vi "Hangup Main.vi"() -> ()   [LabVIEW 2020, in "Hangup Check.lvlib"]
uses:
  Hangup Check.lvlib
  HangupSettings.ctl
  Visualisierungs Elemente/Auswahlfeld.ctl
  AktionFGV Hangup.ctl
  Seiten/FT-IR/FGV FT-IR Gasliste Aktionen.ctl
  Seiten/CalGas Aufschaltung/FGV CalGas Aktionen.ctl
  Sprachverwaltung/FGV Aktion Tabelle zerlegen.ctl
  Messdaten/Aktionen FGV Messdaten.ctl
  Aktion Hangup Test.ctl
  O2 Dichtheitstest/Aktion FGV O2 Leak.ctl
  Funktionstasten/Funktionstasten-Aktion.ctl
  Funktionstasten/Zustaende.ctl
  Seiten/FT-IR/FGV FT-IR Parameter.vi
  Allgemein/allgemeine Sub-VIs.lvlib
  Seiten/FT-IR/FT-IR.lvlib
  Seiten/Grafik/Grafik.lvlib
  Messdaten/Messdaten.lvlib
  Funktionstasten/Funktionstasten.lvlib
  Seiten/CalGas Aufschaltung/CalGas Aufschaltung.lvlib
  O2 Dichtheitstest/O2 Dichtheitstest.lvlib
  Linearisierung V2/Protokoll/Protokoll.lvlib
  Sprachverwaltung/Sprachverwaltung.lvlib
panel:
  out "ppmC1":sgl caption="Ergebnis:" format="%#.1f"
  out "Index":i32
  out "FID":sgl caption="ppmC3" format="%.1f"
  out "Graph CH4":waveform(dbl)(graph)
  out "Bestanden":bool caption="Boolesch"
  out "Zeit":sgl caption="s"
  in  "Textname:":string
  in  "Pfad:":path=path "D:/IAG_Data/Log"
  in  "Speichern":bool
  out "ppmC3":sgl caption="Ergebnis:" format="%#.1f"
  in  "Hangup Settings":T1 {"Grenzwert: C1" format="%#.1f"; "Spankonzentration [ppm]" format="%#.1f"; "Messbereich" items=["---", "0-500", "0-5000", "0-10000"]; "Grenze" items=["Manuell", "Auto"]; "Grenzwert:" format="%#.1f"; "Grenzwert manuell:" format="%#.1f"; "Datenerfassungszeit:" format="%#.1f"; "Nullgas Aufschaltzeit:" format="%#.1f"; "Spangas Aufschaltzeit:" format="%#.1f"; "Aufschaltpunkt" items=["Filterblock", "Analyzer directly", "PNS", "Samplepoint"]; "Kalibriergas" items=["Nitrogen", "Span 1", "Span 2", "Span 3"]}
  in  "Abbrechen":bool
  in  "Test Start":bool
  out "Status":string
  # "Protokoll"
  # "Ergebnis"
  # "Test - Sequenz"
  # "Einstellungen"
  # "Hang-Up-Check"
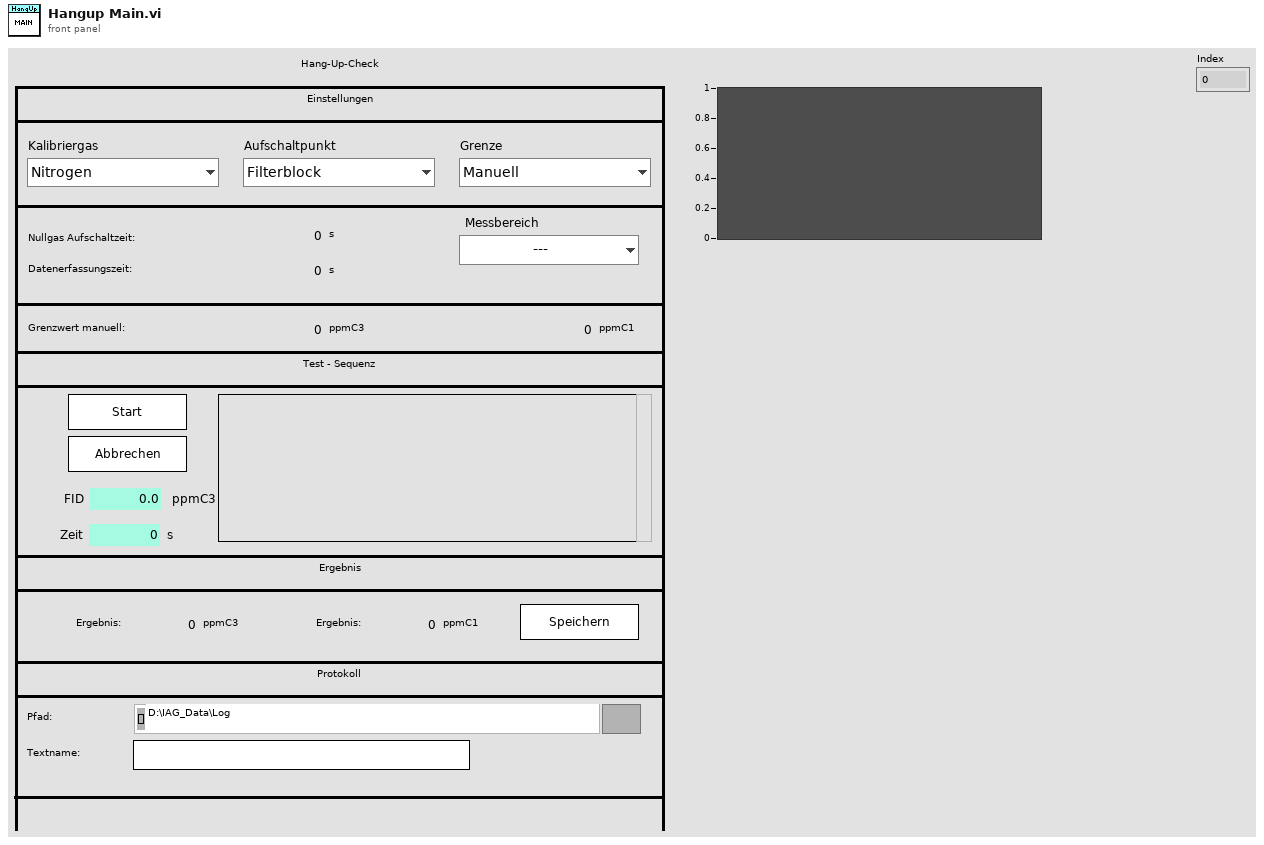
[diagram p1: front panel]
types:
  T1 = typedef "Hangup Check.lvlib/HangupSettings.ctl" = cluster{"Kalibriergas":T2, "Aufschaltpunkt":T2, "Spangas Aufschaltzeit:":sgl, "Nullgas Aufschaltzeit:":sgl, "Datenerfassungszeit:":sgl, "Grenzwert manuell:":sgl, "Grenzwert:":sgl, "Grenze":T2, "Messbereich":T2, "Spankonzentration [ppm]":sgl, "Grenzwert: C1":sgl}
  T2 = typedef "Auswahlfeld.ctl" = u16
  T3 = typedef "Sprachverwaltung.lvlib/FGV Aktion Tabelle zerlegen.ctl" = enum16{"laden", "vereinzeln", "speichern"}
  T4 = typedef "CalGas Aufschaltung.lvlib/FGV CalGas Aktionen.ctl" = enum16{"lesen", "Analysator Auswahl", "Def.CalGas", "Aufschaltung CalGas", "laden", "speichern", "KAL extrahieren"}
  T5 = typedef "FT-IR.lvlib/FGV FT-IR Gasliste Aktionen.ctl" = enum16{"lesen", "Gasliste FT-IR", "Gasliste ausgelesen", "laden", "speichern", "löschen"}
  T6 = enum8{"Enabled", "Disabled", "Disabled and Grayed Out"}
  T7 = typedef "Hangup Check.lvlib/AktionFGV Hangup.ctl" = enum16{"lesen", "Hangup Settings", "Protokoll", "Pfad", "laden", "speichern"}
  T8 = typedef "String - Ausgabefeld.ctl" = string
  T9 = typedef "CalGas Aufschaltung.lvlib/Definition CalGas Anzeige.ctl" = cluster{"Namen":T10, "Werte":T12, "Werte 2":T12, "Einheit":T14, "Messbereiche":T15}
  T10 = typedef "CalGas Aufschaltung.lvlib/CalGas-Namen.ctl" = cluster{"Name":T11, "Name 2":T11, "Name 3":T11, "Name 4":T11, "Name 5":T11, "Name 6":T11, "Name 7":T11, "Name 8":T11, "Name 9":T11, "Name 10":T11, "Name 11":T11, "Name 12":T11}
  T11 = typedef "String - Eingabefeld.ctl" = string
  T12 = typedef "CalGas Aufschaltung.lvlib/CalGas-Werte.ctl" = cluster{"Konzentration 1":T13, "Konzentration 2":T13, "Konzentration 3":T13, "Konzentration 4":T13, "Konzentration 5":T13, "Konzentration 6":T13, "Konzentration 7":T13, "Konzentration 8":T13, "Konzentration 9":T13, "Konzentration 10":T13, "Konzentration 11":T13, "Konzentration 12":T13}
  T13 = typedef "Zahlen-Eingabefeld.ctl" = sgl
  T14 = typedef "CalGas Aufschaltung.lvlib/CalGas-Einheit.ctl" = cluster{"Einheit 1":T2, "Einheit 2":T2, "Einheit 3":T2, "Einheit 4":T2, "Einheit 5":T2, "Einheit 6":T2, "Einheit 7":T2, "Einheit 8":T2, "Einheit 9":T2, "Einheit 10":T2, "Einheit 11":T2, "Einheit 12":T2}
  T15 = typedef "CalGas Aufschaltung.lvlib/CalGas-Messbereiche.ctl" = cluster{"Messbereich 1":T2, "Messbereich 2":T2, "Messbereich 3":T2, "Messbereich 4":T2, "Messbereich 5":T2, "Messbereich 6":T2, "Messbereich 7":T2, "Messbereich 8":T2, "Messbereich 9":T2, "Messbereich 10":T2, "Messbereich 11":T2, "Messbereich 12":T2}
  T16 = typedef "Messdaten.lvlib/Aktionen FGV Messdaten.ctl" = enum16{"lesen", "schreiben", "löschen", "Mittelwerte", "Komponente"}
  T17 = typedef "Hangup Check.lvlib/Aktion Hangup Test.ctl" = enum16{"ini", "0-Gas aufschalten", "warten", "E-Gas aufschalten", "auswerten", "Fertig"}
  T18 = typedef "O2 Dichtheitstest.lvlib/Aktion FGV O2 Leak.ctl" = enum16{"lesen", "O2 settings", "Pfad", "Protokoll", "laden", "speichern"}
  T19 = typedef "Funktionstasten.lvlib/Zustaende.ctl" = enum16{"Standby", "Pause", "Eco", "Messen", "Kalibrieren", "Spülen Filter", "Spülen Leitung", "Umgebungsluft", "0-Gas", "Cal-Gas", "CG zu PNS", "-------------", "Init 1", "Init 2", "Init 3", "Init 4", "Messen vorbereiten", "Messen durchführen", "Exit"}
  T20 = typedef "Funktionstasten.lvlib/Funktionstasten-Aktion.ctl" = enum16{"Initialisieren", "Zustand setzen", "Taste gedrückt", "Fehler speichern", "Lesen", "Manuell", "Remote", "Bitparallel", "Samplepoint", "Zeit Prüfen", "reset Umschalten"}
  T21 = typedef "Hangup Check.lvlib/Protokoll.ctl" = cluster{"FID Mittelwert 0":sgl, "FID Mittelwert E":sgl, "Messgasdruck Amium":sgl, "Startzeit":timestamp, "Endzeit":timestamp, "Bestanden?":bool}
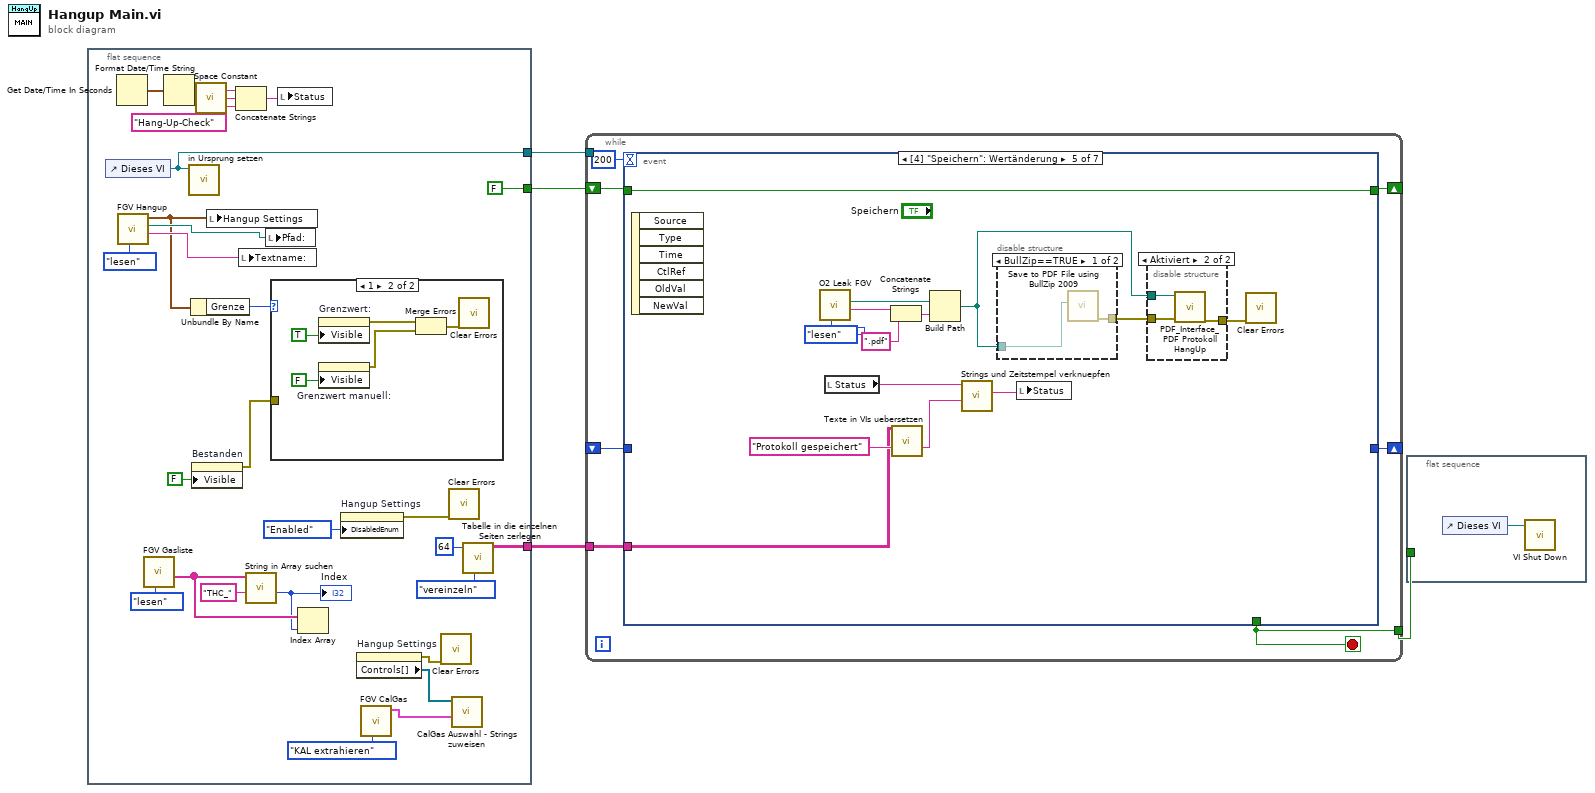
[diagram p0: block diagram]
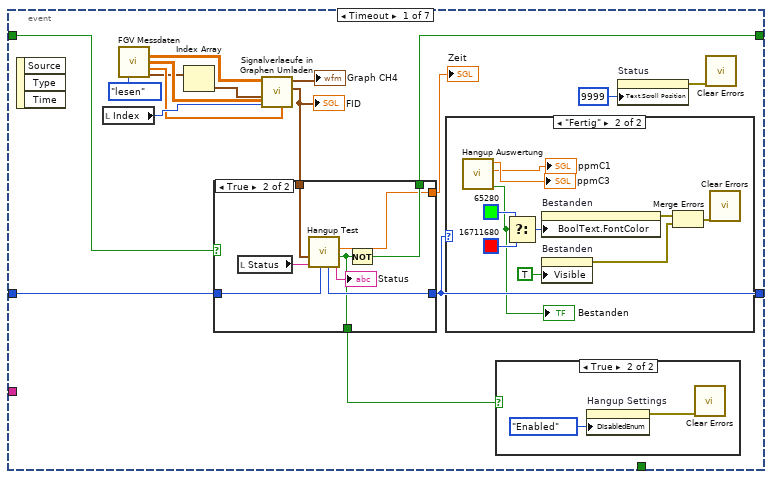
[diagram p2: hidden frame]
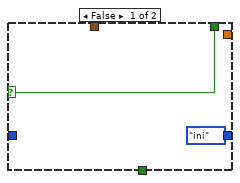
[diagram p5: hidden frame]
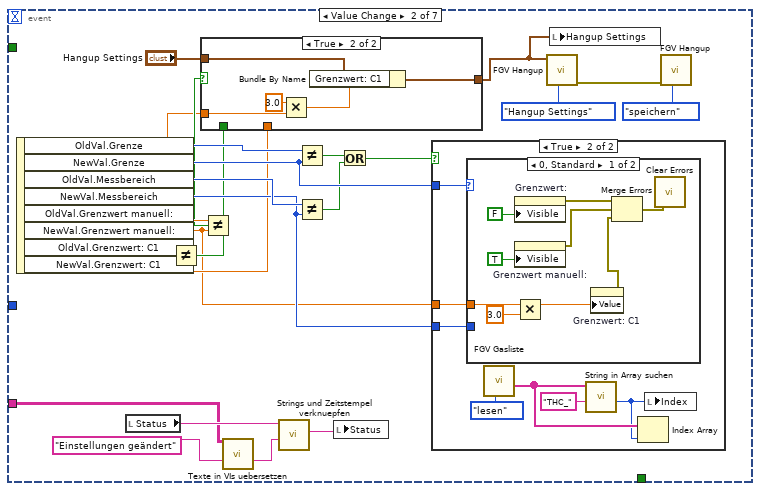
[diagram p6: hidden frame]
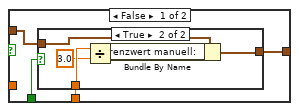
[diagram p7: hidden frame]
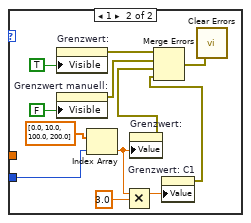
[diagram p10: hidden frame]
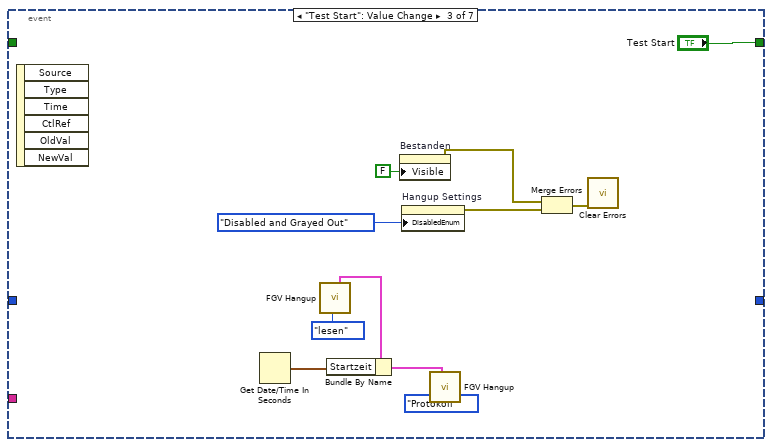
[diagram p11: hidden frame]
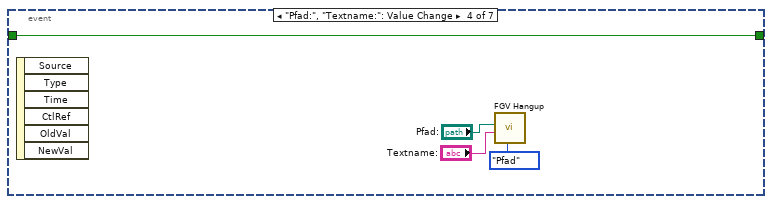
[diagram p12: hidden frame]
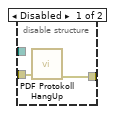
[diagram p13: hidden frame]
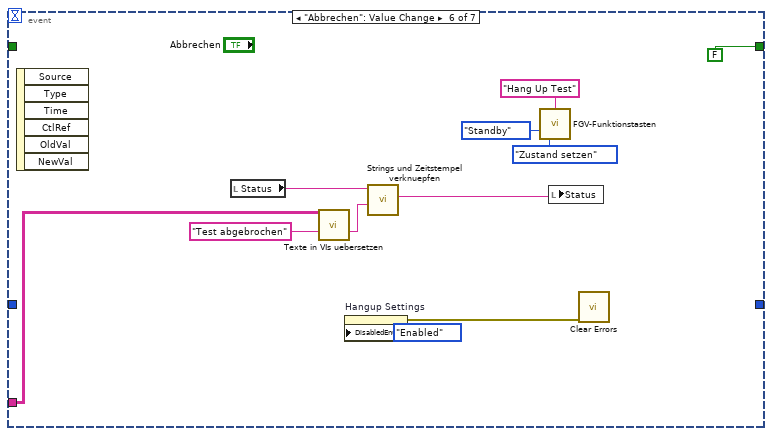
[diagram p15: hidden frame]
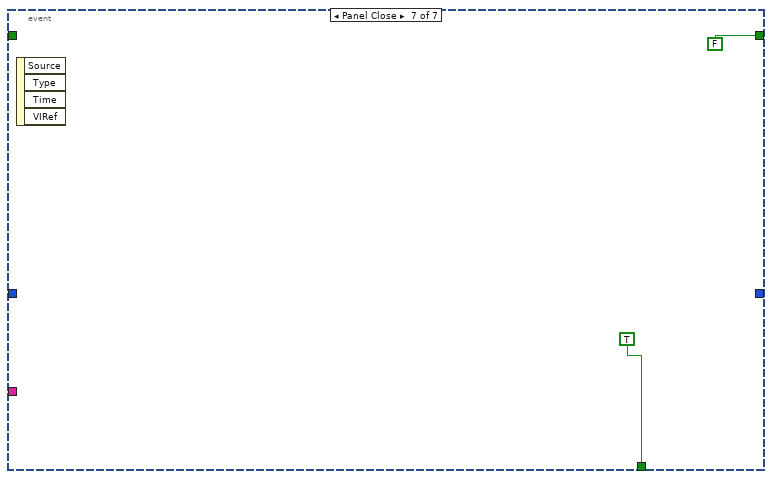
[diagram p16: hidden frame]
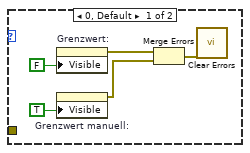
[diagram p17: hidden frame]
diagram:
  n1 = flat-sequence {
    tunnel: [w26] -> w4
    tunnel: [FALSE] -> w2
    tunnel: [w5] -> w1
    frame #0 {
      n2 = control-ref of="Dieses VI"() -> (w26:refnum<vi>)
      n3 = Get Date/Time In Seconds() -> (seconds since 1Jan1904=w22:timestamp)
      n4 = call "FGV Hangup.vi"("Aktion"=AktionFGV_Hangup."lesen") -> ("Textname:"=w29:string, "Pfad:"=w30:path, "Hangup Settings"=w28:T1)  [unwired: 6 in, 2 out]
      n5 = call "FGV Gasliste.vi"("Aktionen"=FGV_FT-IR_Gasliste_Aktionen."lesen") -> ("Aktuelle Gasliste gesamt"=w17:T8[])  [unwired: 8 in, 2 out]
      n6 = Format Date/Time String(seconds (now)=w22) -> (date/time string=w23:string)  [unwired: 2 in]
      n7 = call "in Ursprung setzen.vi"("VI Referenz"=w26) -> ()  [unwired: 10 in, 1 out]
      n8 = Unbundle By Name(w28) -> ("Grenze"=w27:T2)
      n9 = property on="Bestanden" class="Bool. (strikt)"("Visible"=FALSE ("Sichtbar")) -> (error out=w12:errorcluster)  [unwired: 2 in, 1 out]
      n10 = call <vilib>:"Space Constant.vi"() -> ("String"=w24:string)
      n11 = local write "Hangup Settings"(w28) -> ()
      n12 = Concatenate Strings(w23, w24, "Hang-Up-Check" ("String")) -> (w21:string)
      n13 = local write "Textname:"(w29) -> ()
      n14 = call "String in Array suchen.vi"("Nach String/Zeichen suchen (-)"="THC_", "String-Array"=w17) -> ("Index"=w14:i32)  [unwired: 7 in, 2 out]
      "Index" <- w14
      n15 = local write "Pfad:"(w30) -> ()
      n16 = case shown="1" w27 {
        tunnel: w12 -> [_ _]
        frame 0, Default {
          n17 = property on="Grenzwert:" class="DigWert (strikt)"("Visible"=FALSE) -> (error out=w33:errorcluster)  [unwired: 2 in, 1 out]
          n18 = property on="Grenzwert manuell:" class="DigWert (strikt)"("Visible"=TRUE) -> (error out=w32:errorcluster)  [unwired: 2 in, 1 out]
          n19 = Merge Errors(w33, w32) -> (w34:errorcluster)
          n20 = call <vilib>:"Clear Errors.vi"("error in (no error)"=w34) -> ()  [unwired: 5 in, 2 out]
        }
        frame 1 {
          n21 = property on="Grenzwert:" class="DigWert (strikt)"("Visible"=TRUE) -> (error out=w38:errorcluster)  [unwired: 2 in, 1 out]
          n22 = property on="Grenzwert manuell:" class="DigWert (strikt)"("Visible"=FALSE) -> (error out=w37:errorcluster)  [unwired: 2 in, 1 out]
          n23 = Merge Errors(w38, w37) -> (w39:errorcluster)
          n24 = call <vilib>:"Clear Errors.vi"("error in (no error)"=w39) -> ()  [unwired: 5 in, 2 out]
        }
      }
      n25 = local write "Status"(w21) -> ()
      n26 = Index Array(array=w17, index=w14) -> ()  [unwired: 1 out]
      n27 = property on="Hangup Settings" class="Cluster (strikt)"("DisabledEnum"=T6."Enabled" ("Deaktiviert")) -> (error out=w19:errorcluster)  [unwired: 2 in, 1 out]
      n28 = property on="Hangup Settings" class="Cluster (strikt)"() -> (error out=w8:errorcluster, "Controls[]"=w11:refnum<vi>[])  [unwired: 2 in, 1 out]
      n29 = call "FGV CalGas.vi"("Aktionen"=FGV_CalGas_Aktionen."KAL extrahieren") -> ("Def.CalGas"=w10:T9)  [unwired: 6 in, 4 out]
      n30 = call <vilib>:"Clear Errors.vi"("error in (no error)"=w8) -> ()  [unwired: 5 in, 2 out]
      n31 = call <vilib>:"Clear Errors.vi"("error in (no error)"=w19) -> ()  [unwired: 5 in, 2 out]
      n32 = call "CalGas Auswahl - Strings zuweisen.vi"("Def.CalGas"=w10, "Aufschaltung CalGas"=w11) -> ()  [unwired: 9 in, 1 out]
      n33 = call "Tabelle in die einzelnen Seiten zerlegen.vi"("Aktion"=FGV_Aktion_Tabelle_zerlegen."vereinzeln", "Index (Seite)"=64) -> ("Sprachliste"=w5:string[][])  [unwired: 7 in, 2 out]
    }
  }
  n34 = while {
    tunnel: w4 -> [_]
    tunnel: [w48] -> w3
    shift-right: [w47] -> _
    shift-left: w2 -> [w46]
    shift-right: [w44] -> _
    shift-left: _ -> [w43]
    tunnel: w1 -> [w42]
    stop <- w48 stop-if-true
    n35 = event shown="[4] \"Speichern\": Wertänderung" {
      selector: _ -> [_ _ _ _ _ _ _]
      dyn-events: _ -> [_ _ _ _ _ _ _]
      timeout: 200 -> [_ _ _ _ _ _ _]
      tunnel: [_ _ _ _ _ _ TRUE] -> w48
      tunnel: [w61 _ "Test Start" w165 w180 FALSE ("Test Start") FALSE ("Test Start")] -> w47
      tunnel: w46 -> [w63 _ _ w165 w180 _ _]
      tunnel: [w58 _ _ _ _ _ _] -> w44
      tunnel: w43 -> [w62 _ _ _ _ _ _]
      tunnel: w42 -> [_ w88 _ _ w175 w190 _]
      event Timeout {
        n36 = event-data() -> ()  [unwired: 1 in, 3 out]
        n37 = local read "Index"() -> (w57:i32)
        n38 = call "FGV Messdaten.vi"("Aktionen"=Aktionen_FGV_Messdaten."lesen") -> ("Messdaten"=w53:sgl[][], "Mittelwertdaten"=w55:sgl[][], "Deviation"=w56:sgl[], "Zeitstempeln"=w51:timestamp[])  [unwired: 6 in, 5 out]
        n39 = Index Array(array=w51) -> (element=w54:timestamp)  [unwired: 1 in]
        n40 = call "Signalverlaeufe in Graphen Umladen.vi"("Deviation"=w56, "Mittelwertdaten"=w55, "Gas-Auswahl"=w57, "t0"=w54, "Werte"=w53) -> ("Mittelwert"=w49:waveform(dbl), "Waveform"=→"Graph CH4":waveform(dbl))  [unwired: 2 in, 3 out]
        "FID" <- w49
        n41 = case shown="True" w63 {
          selector: w63 -> [w78 _]
          tunnel: [Aktion_Hangup_Test."ini" ("Aktion Hangup Test 2") w87] -> w58
          tunnel: w62 -> [_ w86]
          tunnel: [w78 w85] -> w61
          tunnel: [_ w82] -> w60
          tunnel: [_ w81] -> w59
          tunnel: w49 -> [_ w80]
          frame False {
          }
          frame True {
            n42 = local read "Status"() -> (w83:string)
            n43 = call "Hangup Test.vi"("Aktion Hangup Test"=w86, "Status"=w83, "FID"=w80) -> ("Status"=→"Status":string, "Test beendet?"=w82:bool, "countdonw"=w81:dbl, "Aktion Hangup Test 2"=w87:T17)  [unwired: 5 in]
            n44 = Not(x=w82) -> (.not. x?=w85:bool)
          }
        }
        "Zeit" <- w59
        n45 = case shown="\"Fertig\"" w58 {
          frame "ini", Default {
          }
          frame "Fertig" {
            n46 = call "Hangup Auswertung.vi"() -> ("Bestanden"=w67:bool, "Ergebnis ppmC1 2"=→"ppmC1":sgl, "Ergebnis ppmC3"=→"ppmC3":sgl)  [unwired: 9 in]
            "Bestanden" <- w67
            n47 = Select(t=u32 65280, s=w67, f=u32 16711680) -> (s? t:f=w73:u32)
            n48 = property on="Bestanden" class="Bool. (strikt)"("BoolText.FontColor"=w73) -> (error out=w70:errorcluster)  [unwired: 2 in, 1 out]
            n49 = property on="Bestanden" class="Bool. (strikt)"("Visible"=TRUE ("Sichtbar")) -> (error out=w71:errorcluster)  [unwired: 2 in, 1 out]
            n50 = Merge Errors(w70, w71) -> (w69:errorcluster)
            n51 = call <vilib>:"Clear Errors.vi"("error in (no error)"=w69) -> ()  [unwired: 5 in, 2 out]
          }
        }
        n52 = case shown="True" w60 {
          frame False {
          }
          frame True {
            n53 = property on="Hangup Settings" class="Cluster (strikt)"("DisabledEnum"=T6."Enabled" ("Deaktiviert")) -> (error out=w76:errorcluster)  [unwired: 2 in, 1 out]
            n54 = call <vilib>:"Clear Errors.vi"("error in (no error)"=w76) -> ()  [unwired: 5 in, 2 out]
          }
        }
        n55 = property on="Status" class="Str"("Text.Scroll Position"=u32 9999 ("Text.Anzeigeposition")) -> (error out=w64:errorcluster)  [unwired: 2 in, 1 out]
        n56 = call <vilib>:"Clear Errors.vi"("error in (no error)"=w64) -> ()  [unwired: 5 in, 2 out]
      }
      event Value Change {
        n57 = event-data() -> ("OldVal.Grenze"=w105:T2, "NewVal.Grenze"=w104:T2, "OldVal.Messbereich"=w103:T2, "NewVal.Messbereich"=w99:T2, "OldVal.Grenzwert manuell:"=w98:sgl, "NewVal.Grenzwert manuell:"=w91:sgl, "OldVal.Grenzwert: C1"=w97:sgl, "NewVal.Grenzwert: C1"=w93:sgl)  [unwired: 1 in]
        n58 = local read "Status"() -> (w107:string)
        n59 = Not Equal?(x=w97, y=w93) -> (x != y?=w94:bool)
        n60 = Not Equal?(x=w98, y=w91) -> (x != y?=w95:bool)
        n61 = case shown="True" w95 {
          tunnel: "Hangup Settings" -> [w112 w125]
          tunnel: [w111 w124] -> w92
          tunnel: w91 -> [_ w123]
          tunnel: w94 -> [w114 _]
          tunnel: w93 -> [w113 _]
          frame False {
            n62 = case shown="True" w114 {
              tunnel: w113 -> [_ w120]
              tunnel: w112 -> [w115 w117]
              tunnel: [w115 w116] -> w111
              frame False {
              }
              frame True {
                n63 = Divide(x=w120, y=sgl 3.0) -> (x/y=w118:sgl)
                n64 = Bundle By Name(cluster=w117, "Grenzwert manuell:"=w118) -> (w116:T1)
              }
            }
          }
          frame True {
            n65 = Multiply(x=sgl 3.0, y=w123) -> (x*y=w121:sgl)
            n66 = Bundle By Name(cluster=w125, "Grenzwert: C1"=w121) -> (w124:T1)
          }
        }
        n67 = call "Texte in VIs uebersetzen.vi"("Sprachliste"=w88, "String zum Übersetzen"="Einstellungen geändert" ("String 1 hinzufügen")) -> ("String zum Übersetzen"=w89:string)  [unwired: 9 in, 4 out]
        n68 = call "Strings und Zeitstempel verknuepfen.vi"("String 1 hinzufügen"=w89, "Eingagns String"=w107) -> ("Verknüpfter String"=w106:string)  [unwired: 9 in]
        n69 = Not Equal?(x=w105, y=w104) -> (x != y?=w102:bool)
        n70 = Not Equal?(x=w103, y=w99) -> (x != y?=w101:bool)
        n71 = local write "Status"(w106) -> ()
        n72 = Or(x=w102, y=w101) -> (x .or. y?=w100:bool)
        n73 = case shown="True" w100 {
          tunnel: w104 -> [_ w132]
          tunnel: w99 -> [_ w127]
          tunnel: w91 -> [_ w126]
          frame False {
          }
          frame True {
            n74 = case shown="0, Standard" w132 {
              tunnel: w127 -> [_ w146]
              tunnel: w126 -> [w135 _]
              frame 0, Default {
                n75 = property on="Grenzwert:" class="DigWert (strikt)"("Visible"=FALSE) -> (error out=w138:errorcluster)  [unwired: 2 in, 1 out]
                n76 = property on="Grenzwert manuell:" class="DigWert (strikt)"("Visible"=TRUE) -> (error out=w137:errorcluster)  [unwired: 2 in, 1 out]
                n77 = Multiply(x=w135, y=sgl 3.0) -> (x*y=w134:sgl)
                n78 = property on="Grenzwert: C1" class="DigWert (strikt)"("Value"=w134) -> (error out=w136:errorcluster)  [unwired: 2 in, 1 out]
                n79 = Merge Errors(w138, w137, w136) -> (w139:errorcluster)
                n80 = call <vilib>:"Clear Errors.vi"("error in (no error)"=w139) -> ()  [unwired: 5 in, 2 out]
              }
              frame 1 {
                n81 = property on="Grenzwert:" class="DigWert (strikt)"("Visible"=TRUE) -> (error out=w150:errorcluster)  [unwired: 2 in, 1 out]
                n82 = property on="Grenzwert manuell:" class="DigWert (strikt)"("Visible"=FALSE) -> (error out=w149:errorcluster)  [unwired: 2 in, 1 out]
                n83 = Index Array(array=sgl[] [0.0, 10.0, 100.0, 200.0] ("Wert"), index=w146) -> (element=w145:sgl)
                n84 = Multiply(x=w145, y=sgl 3.0) -> (x*y=w144:sgl)
                n85 = property on="Grenzwert:" class="DigWert (strikt)"("Value"=w145) -> (error out=w148:errorcluster)  [unwired: 2 in, 1 out]
                n86 = property on="Grenzwert: C1" class="DigWert (strikt)"("Value"=w144) -> (error out=w142:errorcluster)  [unwired: 2 in, 1 out]
                n87 = Merge Errors(w150, w149, w148, w142) -> (w151:errorcluster)
                n88 = call <vilib>:"Clear Errors.vi"("error in (no error)"=w151) -> ()  [unwired: 5 in, 2 out]
              }
            }
            n89 = call "FGV Gasliste.vi"("Aktionen"=FGV_FT-IR_Gasliste_Aktionen."lesen") -> ("Aktuelle Gasliste gesamt"=w129:T8[])  [unwired: 8 in, 2 out]
            n90 = call "String in Array suchen.vi"("Nach String/Zeichen suchen (-)"="THC_", "String-Array"=w129) -> ("Index"=w128:i32)  [unwired: 7 in, 2 out]
            n91 = Index Array(array=w129, index=w128) -> ()  [unwired: 1 out]
            n92 = local write "Index"(w128) -> ()
          }
        }
        n93 = call "FGV Hangup.vi"("Aktion"=AktionFGV_Hangup."Hangup Settings", "Hangup Settings"=w92) -> ("error out"=w108:errorcluster)  [unwired: 5 in, 4 out]
        n94 = local write "Hangup Settings"(w92) -> ()
        n95 = call "FGV Hangup.vi"("Aktion"=AktionFGV_Hangup."speichern", "error in (no error)"=w108) -> ()  [unwired: 5 in, 5 out]
      }
      event "Test Start": Value Change {
        n96 = event-data() -> ()  [unwired: 1 in, 6 out]
        n97 = Get Date/Time In Seconds() -> (seconds since 1Jan1904=w157:timestamp)
        n98 = call "FGV Hangup.vi"("Aktion"=AktionFGV_Hangup."lesen") -> ("Protokoll"=w159:T21)  [unwired: 6 in, 4 out]
        n99 = Bundle By Name(cluster=w159, "Startzeit"=w157) -> (w161:T21)
        n100 = property on="Bestanden" class="Bool. (strikt)"("Visible"=FALSE ("Sichtbar")) -> (error out=w154:errorcluster)  [unwired: 2 in, 1 out]
        n101 = property on="Hangup Settings" class="Cluster (strikt)"("DisabledEnum"=T6."Disabled and Grayed Out" ("Deaktiviert")) -> (error out=w162:errorcluster)  [unwired: 2 in, 1 out]
        n102 = call "FGV Hangup.vi"("Aktion"=AktionFGV_Hangup."Protokoll", "Protokoll"=w161) -> ()  [unwired: 5 in, 5 out]
        n103 = Merge Errors(w154, w162) -> (w155:errorcluster)
        n104 = call <vilib>:"Clear Errors.vi"("error in (no error)"=w155) -> ()  [unwired: 5 in, 2 out]
      }
      event "Pfad:", "Textname:": Value Change {
        n105 = event-data() -> ()  [unwired: 1 in, 6 out]
        n106 = call "FGV Hangup.vi"("Aktion"=AktionFGV_Hangup."Pfad", "Textname:"="Textname:", "Pfad:"="Pfad:") -> ()  [unwired: 4 in, 5 out]
      }
      event "Speichern": Value Change {
        n107 = event-data() -> ()  [unwired: 1 in, 6 out]
        n108 = call "O2 Leak FGV.vi"("Aktion"=Aktion_FGV_O2_Leak."lesen") -> ("Textname:"=w173:string, "Pfad:"=w174:path)  [unwired: 6 in, 3 out]
        n109 = local read "Status"() -> (w182:string)
        n110 = Concatenate Strings(w173, ".pdf") -> (w172:string)
        n111 = call "Texte in VIs uebersetzen.vi"("Sprachliste"=w175, "String zum Übersetzen"="Protokoll gespeichert" ("String 1 hinzufügen")) -> ("String zum Übersetzen"=w176:string)  [unwired: 9 in, 4 out]
        n112 = Build Path(base path=w174, name or relative path=w172) -> (appended path=w169:path)
        n113 = call "Strings und Zeitstempel verknuepfen.vi"("String 1 hinzufügen"=w176, "Eingagns String"=w182) -> ("Verknüpfter String"=w181:string)  [unwired: 9 in]
        n114 = disable-structure shown="BullZip==TRUE" {
          disable-tunnel: [w189 _] -> w178
          disable-tunnel: w169 -> [w188 _]
          frame condition #0 {
            n115 = call "Save to PDF File using BullZip 2009.vi"("Save PDF File Path"=w188) -> ("error out"=w189:errorcluster)  [unwired: 10 in]
          }
          frame condition #1 (active) {
          }
        }
        n116 = local write "Status"(w181) -> ()
        n117 = disable-structure shown="Aktiviert" {
          disable-tunnel: [w184 w186] -> w179
          disable-tunnel: w178 -> [w183 w187]
          disable-tunnel: w169 -> [_ w185]
          frame Disabled {
            n118 = call "PDF Protokoll HangUp.vi"("error in (no error)"=w183) -> ("error out"=w184:errorcluster)  [unwired: 10 in]
          }
          frame Enabled {
            n119 = call "PDF_Interface_PDF Protokoll HangUp.vi"("error in (no error)"=w187, "Save PDF File Path"=w185) -> ("error out"=w186:errorcluster)  [unwired: 9 in]
          }
        }
        n120 = call <vilib>:"Clear Errors.vi"("error in (no error)"=w179) -> ()  [unwired: 5 in, 2 out]
      }
      event "Abbrechen": Value Change {
        n121 = event-data() -> ()  [unwired: 1 in, 6 out]
        n122 = local read "Status"() -> (w199:string)
        n123 = call "Texte in VIs uebersetzen.vi"("Sprachliste"=w190, "String zum Übersetzen"="Test abgebrochen" ("String 1 hinzufügen")) -> ("String zum Übersetzen"=w191:string)  [unwired: 9 in, 4 out]
        n124 = property on="Hangup Settings" class="Cluster (strikt)"("DisabledEnum"=T6."Enabled" ("Deaktiviert")) -> (error out=w196:errorcluster)  [unwired: 2 in, 1 out]
        n125 = call "Strings und Zeitstempel verknuepfen.vi"("String 1 hinzufügen"=w191, "Eingagns String"=w199) -> ("Verknüpfter String"=w198:string)  [unwired: 9 in]
        n126 = call "FGV-Funktionstasten.vi"("Herkunft"="Hang Up Test", "Zustand"=Zustaende."Standby", "Aktion"=Funktionstasten-Aktion."Zustand setzen") -> ()  [unwired: 5 in, 8 out]
        n127 = local write "Status"(w198) -> ()
        n128 = call <vilib>:"Clear Errors.vi"("error in (no error)"=w196) -> ()  [unwired: 5 in, 2 out]
      }
      event Panel Close {
        n129 = event-data() -> ()  [unwired: 1 in, 4 out]
      }
    }
  }
  n130 = flat-sequence {
    tunnel: w3 -> [_]
    frame #0 {
      n131 = control-ref of="Dieses VI"() -> (w203:refnum<vi>)
      n132 = call "VI Shut Down.vi"("VI Referenz"=w203) -> ()  [unwired: 11 in]
    }
  }
